vi "SetCh.vi"(0 "MagiQmw3 in":refnum<class "MagiQmw3.lvclass">, 2 "ch":i32, 7 "freq":dbl, 9 "atten":dbl, 11 "error in (no error)":errorcluster) -> (4 "MagiQmw3 out":refnum<class "MagiQmw3.lvclass">, 15 "error out":errorcluster)   [LabVIEW 2010, in "MagiQmw3.lvclass"]
uses:
  MagiQmw3.lvclass
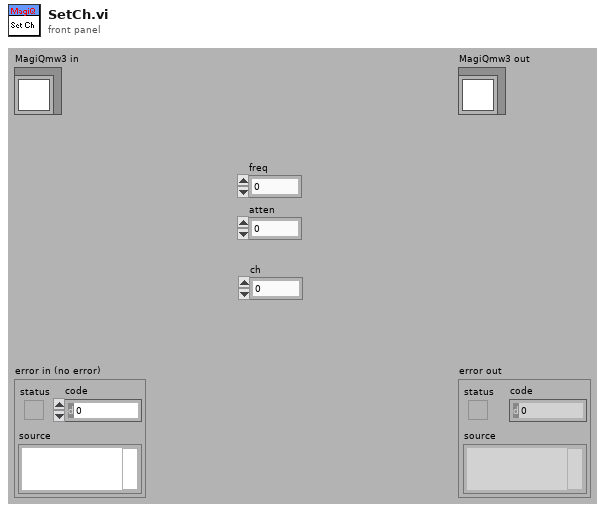
[diagram p1: front panel]
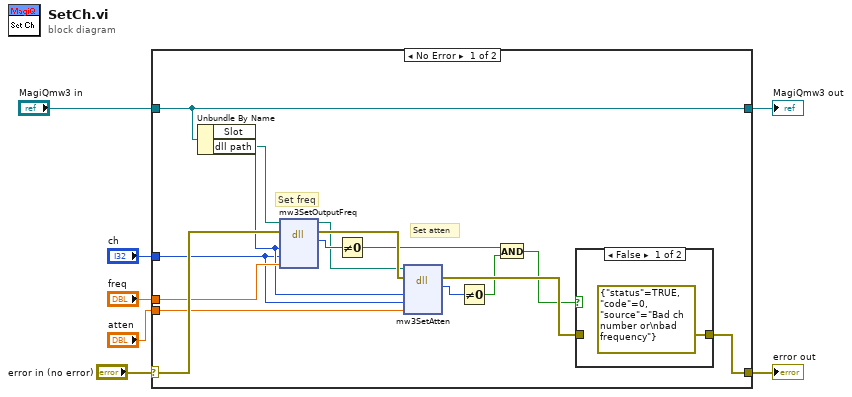
[diagram p0: block diagram]
diagram:
  n1 = case shown="No Error" "error in (no error)" {
    selector: "error in (no error)" -> [w22 w27]
    tunnel: [w21 w27] -> w7
    tunnel: [w23 w26] -> w5
    tunnel: "MagiQmw3 in" -> [w23 w26]
    tunnel: "ch" -> [w14 _]
    tunnel: "freq" -> [w20 _]
    tunnel: "atten" -> [w16 _]
    frame No Error {
      # "Set atten"
      # "Set freq"
      n2 = Unbundle By Name(w23) -> ("Slot"=w15:u16, "dll path"=w9:path)
      n3 = dll-call lib="PulserLib.dll" fn="mw3SetOutputFreq"(path in=w9, error in=w22, "slot"=w15, "ch"=w14, "freq"=w20) -> (path out=w8:path, error out=w18:errorcluster, "return"=w19:i32)  [unwired: 4 in]
      n4 = Not Equal To 0?(x=w19) -> (x != 0?=w11:bool)
      n5 = dll-call lib="PulserLib.dll" fn="mw3SetAtten"(path in=w8, error in=w18, "slot"=w15, "ch"=w14, "loss"=w16) -> (error out=w17:errorcluster, "return"=w13:i32)  [unwired: 4 in, 1 out]
      n6 = Not Equal To 0?(x=w13) -> (x != 0?=w12:bool)
      n7 = And(x=w11, y=w12) -> (x .and. y?=w10:bool)
      n8 = case shown="False" w10 {
        tunnel: [errorcluster {"status"=TRUE, "code"=0, "source"="Bad ch number or\nbad frequency"} ("error in (no error)") w25] -> w21
        tunnel: w17 -> [_ w25]
        frame False {
        }
        frame True {
        }
      }
    }
    frame Error {
    }
  }
  "error out" <- w7
  "MagiQmw3 out" <- w5
